vi "Spawned VI (reentrant).vi"() -> (2 "Count":i32(slide) scale=0.0..100.0)   [LabVIEW 2011]
panel:
  in  "stop":bool
  # "This VI is reentrant.\nThis VI will run until Count reaches 100 or if the user presses the Stop button"
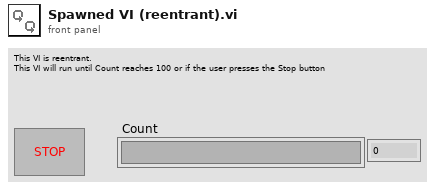
[diagram p1: front panel]
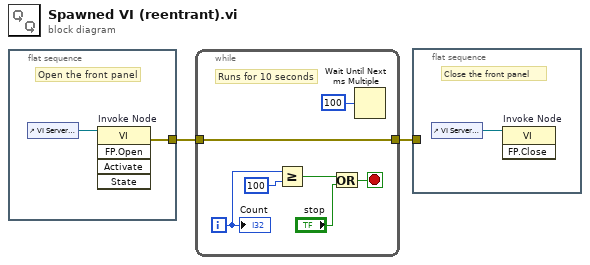
[diagram p0: block diagram]
diagram:
  n1 = flat-sequence {
    tunnel: [w3] -> w2
    frame #0 {
      # "Open the front panel"
      n2 = control-ref of="VI Server Reference"() -> (w4:refnum<vi>)
      n3 = invoke on="Invoke Node" class="VI" method="FP.Open"(reference=w4) -> (error out=w3:errorcluster)  [unwired: 4 in, 4 out]
    }
  }
  n4 = while {
    tunnel: w2 -> [w5]
    tunnel: [w5] -> w1
    i -> [w8]
    stop <- w6 stop-if-true
    # "Runs for 10 seconds"
    n5 = Greater Or Equal?(x=w8, y=100) -> (x >= y?=w7:bool)
    n6 = Or(x=w7, y="stop") -> (x .or. y?=w6:bool)
    n7 = Wait Until Next ms Multiple(millisecond multiple=u32 100) -> ()  [unwired: 1 out]
    "Count" <- w8
  }
  n8 = flat-sequence {
    tunnel: w1 -> [_]
    frame #0 {
      # "Close the front panel"
      n9 = control-ref of="VI Server Reference"() -> (w12:refnum<vi>)
      n10 = invoke on="Invoke Node" class="VI" method="FP.Close"(reference=w12) -> ()  [unwired: 2 in, 3 out]
    }
  }
